vi "RescanUSB.vi"(0 "COM":string, 1 "TimeOut For Scanning":u32, 11 "error in (no error)":errorcluster) -> (3 "succes?":bool, 15 "error out":errorcluster)   [LabVIEW 2014]
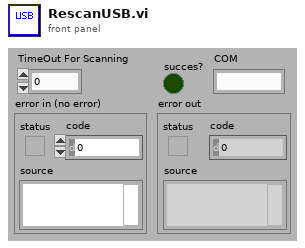
[diagram p1: front panel]
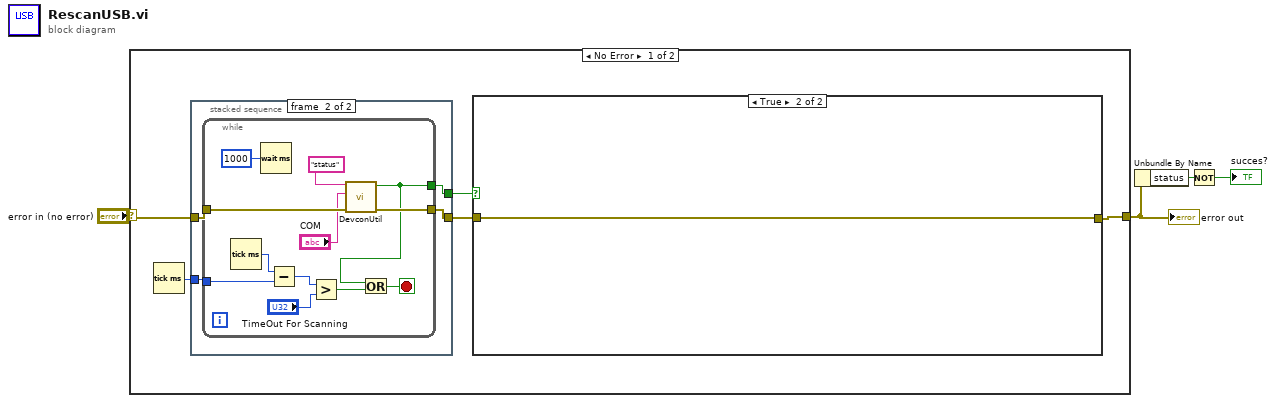
[diagram p0: block diagram]
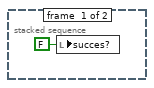
[diagram p2: hidden frame]
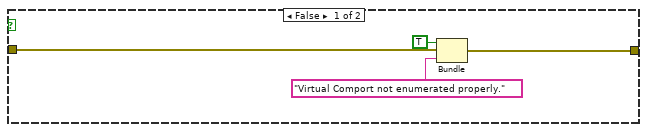
[diagram p3: hidden frame]
diagram:
  n1 = case shown="No Error" "error in (no error)" {
    selector: "error in (no error)" -> [w9 w32]
    tunnel: [w6 w32] -> w3
    frame No Error {
      n2 = Tick Count (ms)() -> (millisecond timer value=w5:u32)
      n3 = stacked-sequence {
        tunnel: w9 -> [_ w14]
        tunnel: [_ w13] -> w8
        tunnel: [_ w12] -> w7
        tunnel: w5 -> [_ w11]
        frame #0 {
          n4 = local write "succes?"(FALSE ("succes?")) -> ()
        }
        frame #1 {
          n5 = while {
            tunnel: w14 -> [w25]
            tunnel: [w18] -> w13
            tunnel: [w24] -> w12
            tunnel: w11 -> [w22]
            stop <- w20 stop-if-true
            n6 = Tick Count (ms)() -> (millisecond timer value=w23:u32)
            n7 = Wait (ms)(milliseconds to wait=u32 1000) -> ()  [unwired: 1 out]
            n8 = Subtract(x=w23, y=w22) -> (x-y=w17:u32)
            n9 = Greater?(x=w17, y="TimeOut For Scanning") -> (0:w19:bool)
            n10 = call "DevconUtil.vi"("error in (no error)"=w25, "COM"="COM", "Action"="status") -> ("error out"=w24:errorcluster, "success?"=w18:bool)  [unwired: 4 in, 1 out]
            n11 = Or(x=w18, y=w19) -> (x .or. y?=w20:bool)
          }
        }
      }
      n12 = case shown="True" w8 {
        tunnel: w7 -> [w30 w31]
        tunnel: [w28 w31] -> w6
        frame False {
          n13 = Bundle(cluster=w30, "status"=TRUE, "source"="Virtual Comport not enumerated properly.") -> (w28:errorcluster)  [unwired: 1 in]
        }
        frame True {
        }
      }
    }
    frame Error {
    }
  }
  "error out" <- w3
  n14 = Unbundle By Name(w3) -> ("status"=w2:bool)
  n15 = Not(x=w2) -> (.not. x?=→"succes?":bool)
